vi "Example Morse Code.vi"() -> ()   [LabVIEW 2010]
uses:
  C:/tf/play/labview/Tinkerforge.dll
panel:
  in  "uid":string="amb"
  in  "port":i32=4223
  in  "host":string="localhost"
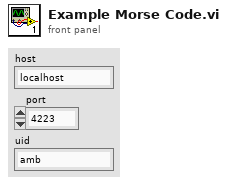
[diagram p1: front panel]
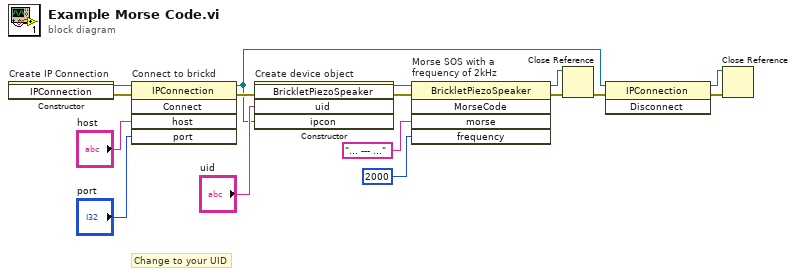
[diagram p0: block diagram]
diagram:
  # "Change to your UID"
  n1 = constructor on="Create IP Connection" class="IPConnection"() -> (reference out=w16:refnum<k24>, error out=w3:errorcluster)  [unwired: 3 in, 1 out]
  n2 = invoke on="Connect to brickd" class="IPConnection" method="Connect"(reference=w16, error in=w3, "host"="host", "port"="port") -> (reference out=w5:refnum<k24>, error out=w12:errorcluster)  [unwired: 1 in, 3 out]
  n3 = constructor on="Create device object" class="BrickletPiezoSpeaker"(error in=w12, "uid"="uid", "ipcon"=w5) -> (reference out=w10:refnum<k24>, error out=w11:errorcluster)  [unwired: 2 in, 3 out]
  n4 = invoke on="Morse SOS with a\nfrequency of 2kHz" class="BrickletPiezoSpeaker" method="MorseCode"(reference=w10, error in=w11, "morse"="... --- ...", "frequency"=2000) -> (reference out=w8:refnum<k24>, error out=w9:errorcluster)  [unwired: 1 in, 3 out]
  n5 = Close Reference(reference=w8, error in (no error)=w9) -> (error out=w7:errorcluster)
  n6 = invoke class="IPConnection" method="Disconnect"(reference=w5, error in=w7) -> (reference out=w4:refnum<k24>, error out=w6:errorcluster)  [unwired: 1 in, 1 out]
  n7 = Close Reference(reference=w4, error in (no error)=w6) -> ()  [unwired: 1 out]
